vi "tempo_map.get.vi"(8 "error in (no error)":errorcluster, 11 "midi-file-events in":refnum<class "midi-file-events.lvclass">) -> (0 "error out":errorcluster, 2 "Tempo Map":map{dbl, dbl}(c390), 3 "midi-file-events out":refnum<class "midi-file-events.lvclass">)   [LabVIEW 2020, in "midi-file-events.lvclass"]
uses:
  midi-file-events.lvclass
  midi-file-events.lvclass/midi-file-events.ctl
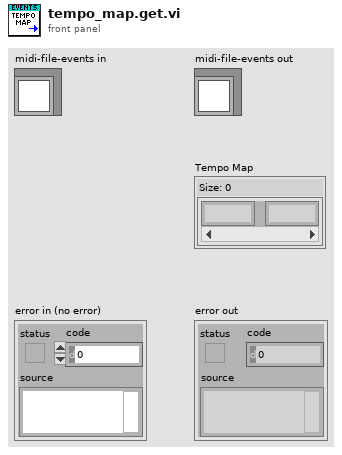
[diagram p1: front panel]
types:
  T1 = typedef "midi-file-events.lvclass/privatedata.ctl" = cluster{"ticks per quarter note (division)":i16, "Tempo Map":map{dbl, dbl}, "Track data by Track number":map{i32, map{dbl, set{refnum<class "midi-file-event.midi.lvclass">}}}}
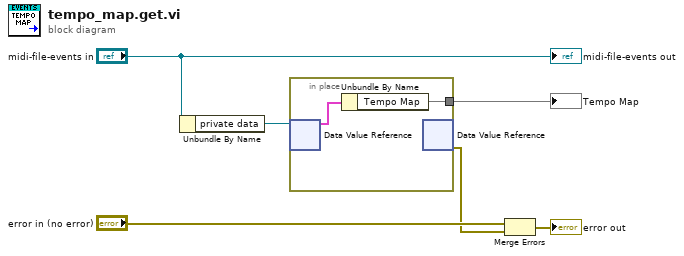
[diagram p0: block diagram]
diagram:
  n1 = Unbundle By Name("midi-file-events in") -> ("private data"=w6:refnum<data-value>)
  n2 = in-place {
    in-place-border: [w7] -> w5
    n3 = in-place-dvr #1(w6) -> (w8:T1)  [unwired: 1 out]
    n4 = Unbundle By Name(w8) -> ("Tempo Map"=w7:map{dbl, dbl})
    n5 = in-place-dvr #1() -> (w2:errorcluster)  [unwired: 1 in, 1 out]
  }
  "Tempo Map" <- w5
  n6 = Merge Errors("error in (no error)", w2) -> (→"error out":errorcluster)
  "midi-file-events out" <- "midi-file-events in"
